vi "Group Terminals.vi"(9 "Terminal Configs":T3[](array[typedef]), 10 "Terminals":refnum<vi>[](array[refnum])) -> (3 "Grouped Terminals":T1)   [LabVIEW 2020, in "FlexBlocks.lvlib"]
uses:
  FlexBlocks.lvlib
  Terminal Config.ctl
  Type Descriptor.ctl
  Terminal Direction.ctl
  Value Mode.ctl
  Special Terminal.ctl
  Terminal Mode.ctl
  Terminal Group.ctl
  Grouped Terminals.ctl
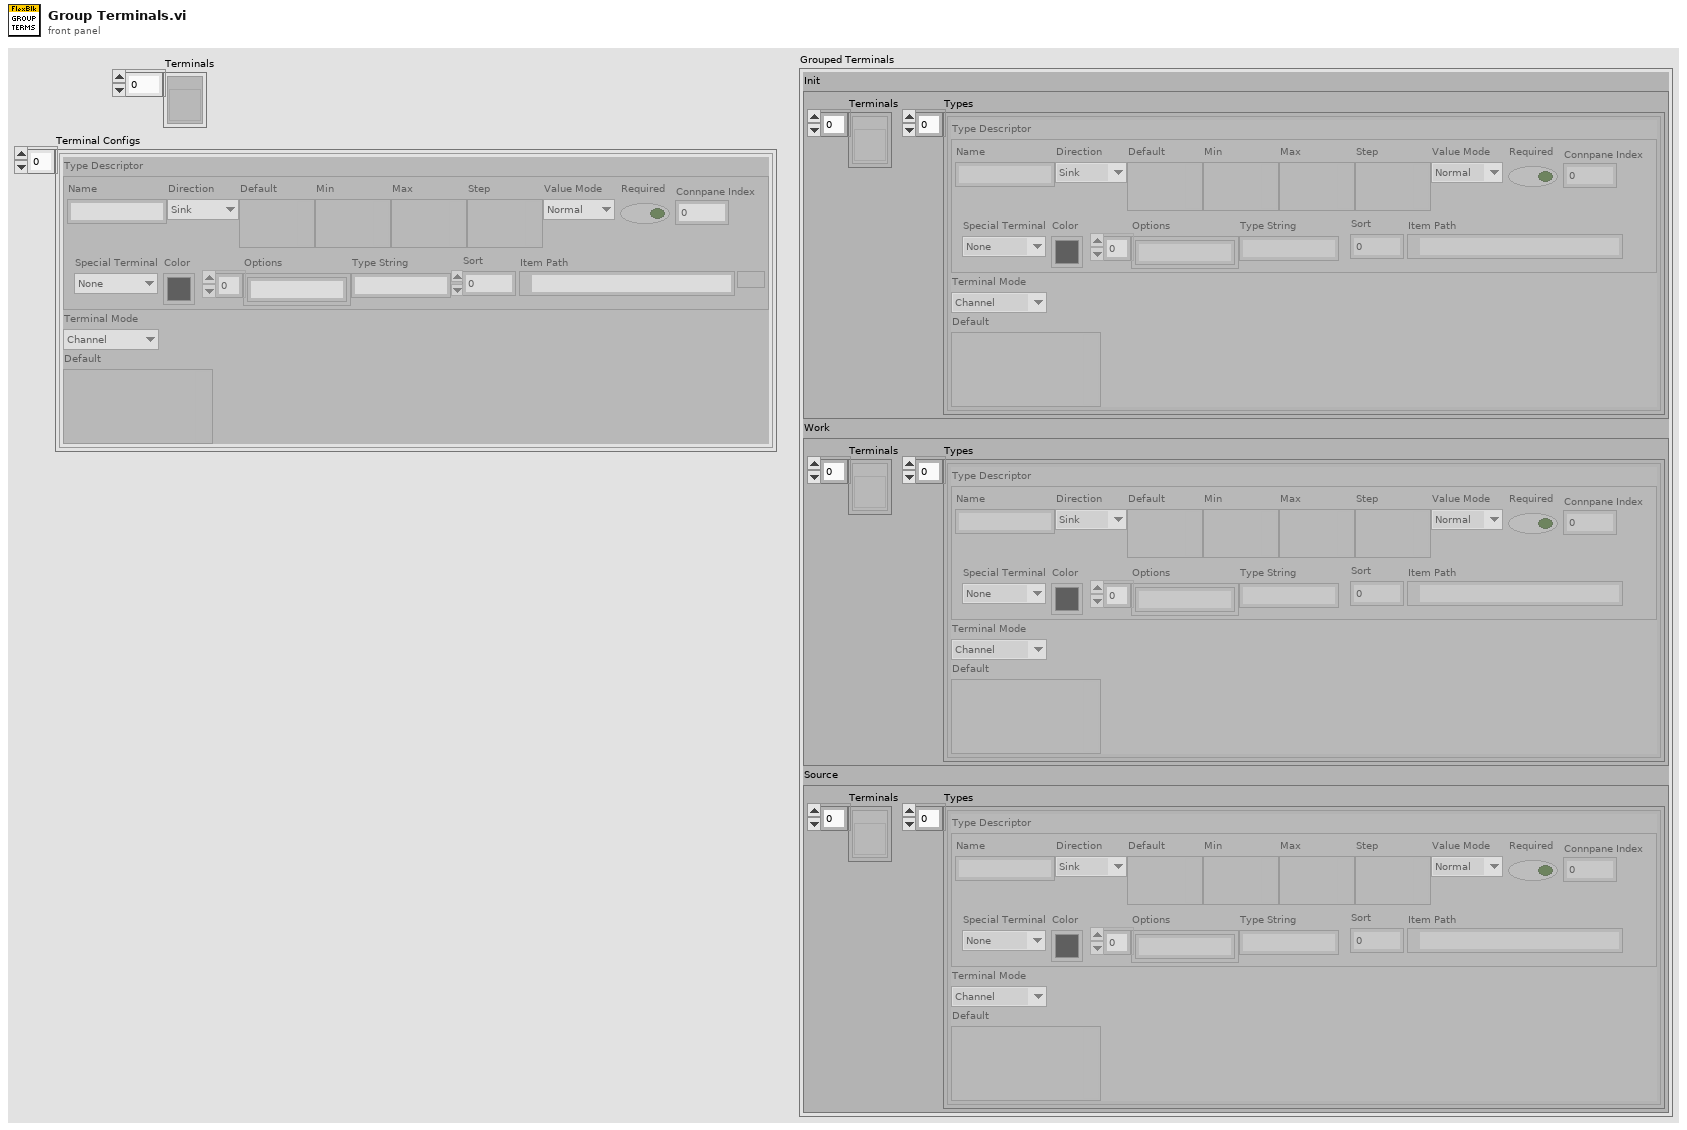
[diagram p1: front panel]
types:
  T1 = typedef "FlexBlocks.lvlib/Grouped Terminals.ctl" = cluster{"Init":T2, "Work":T2, "Source":T2}
  T2 = typedef "FlexBlocks.lvlib/Terminal Group.ctl" = cluster{"Terminals":refnum<vi>[], "Types":T3[]}
  T3 = typedef "FlexBlocks.lvlib/Terminal Config.ctl" = cluster{"Type Descriptor":T4, "Terminal Mode":T8, "Default":variant}
  T4 = typedef "FlexBlocks.lvlib/Type Descriptor.ctl" = cluster{"Name":string, "Direction":T5, "Default":variant, "Min":variant, "Max":variant, "Step":variant, "Value Mode":T6, "Required":bool, "Connpane Index":i32, "Special Terminal":T7, "Color":u32, "Options":string[], "Type String":string, "Sort":i32, "Item Path":path}
  T5 = typedef "FlexBlocks.lvlib/Terminal Direction.ctl" = enum16{"Sink", "Source"}
  T6 = typedef "FlexBlocks.lvlib/Value Mode.ctl" = enum16{"Normal", "Range", "Select"}
  T7 = typedef "FlexBlocks.lvlib/Special Terminal.ctl" = enum16{"None", "Action", "Init", "Tag", "State in", "State out", "Error"}
  T8 = typedef "FlexBlocks.lvlib/Terminal Mode.ctl" = enum16{"Channel", "Config", "Value", "Control Ref"}
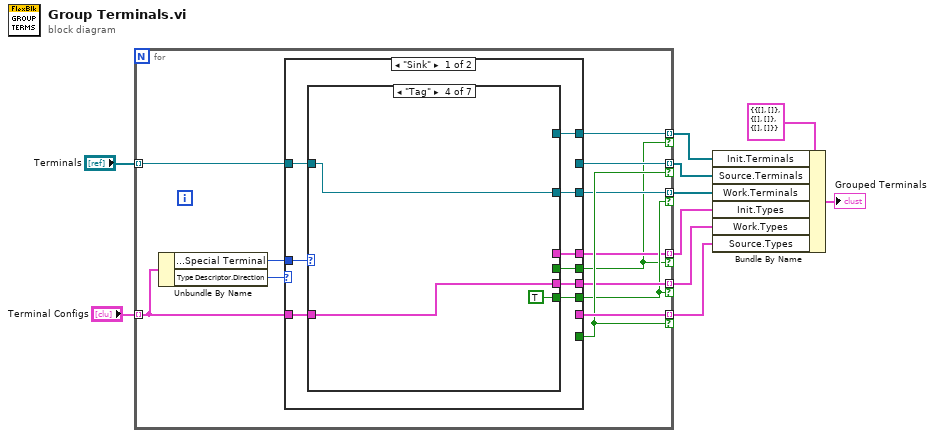
[diagram p0: block diagram]
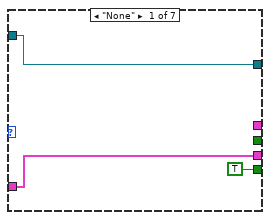
[diagram p2: hidden frame]
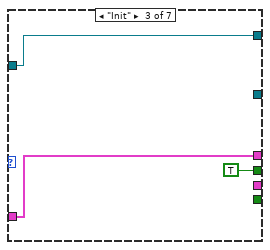
[diagram p4: hidden frame]
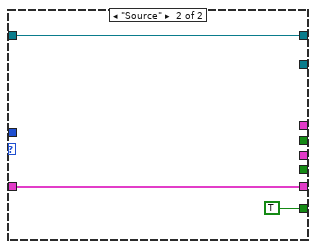
[diagram p8: hidden frame]
diagram:
  n1 = for {
    tunnel: "Terminals" -> [w11] mode=indexing
    tunnel: "Terminal Configs" -> [w21] mode=indexing
    tunnel: [w20] -> w4 mode=indexing if=w18
    tunnel: [w19] -> w3 mode=indexing if=w18
    tunnel: [w17] -> w5 mode=indexing if=w15
    tunnel: [w16] -> w7 mode=indexing if=w15
    tunnel: [w14] -> w2 mode=indexing if=w12
    tunnel: [w13] -> w6 mode=indexing if=w12
    n2 = Unbundle By Name(w21) -> ("Type Descriptor.Special Terminal"=w22:T7, "Type Descriptor.Direction"=w23:T5)
    n3 = case shown="\"Sink\"" w23 {
      tunnel: w22 -> [w32 _]
      tunnel: w11 -> [w31 w42]
      tunnel: w21 -> [w30 w44]
      tunnel: [_ w44] -> w20
      tunnel: [_ TRUE] -> w18
      tunnel: [_ w42] -> w19
      tunnel: [w29 _] -> w17
      tunnel: [w28 _] -> w16
      tunnel: [w27 _] -> w15
      tunnel: [w26 _] -> w14
      tunnel: [w25 _] -> w13
      tunnel: [w24 _] -> w12
      frame "Sink" {
        n4 = case shown="\"Tag\"" w32 {
          tunnel: w31 -> [w34 _ w38 w41 _ _ _]
          tunnel: w30 -> [w35 _ w37 w39 _ _ _]
          tunnel: [w35 _ _ w39 _ _ _] -> w29
          tunnel: [w34 _ _ w41 _ _ _] -> w28
          tunnel: [TRUE _ _ TRUE _ _ _] -> w27
          tunnel: [_ _ w38 _ _ _ _] -> w26
          tunnel: [_ _ w37 _ _ _ _] -> w25
          tunnel: [_ _ TRUE _ _ _ _] -> w24
          frame "None" {
          }
          frame "Action" {
          }
          frame "Init" {
          }
          frame "Tag" {
          }
          frame "State in" {
          }
          frame "State out" {
          }
          frame "Error" {
          }
        }
      }
      frame "Source" {
      }
    }
  }
  n5 = Bundle By Name(cluster=T1 {"Init"={"Terminals"=[], "Types"=[]}, "Work"={"Terminals"=[], "Types"=[]}, "Source"={"Terminals"=[], "Types"=[]}} ("Grouped Terminals"), "Init.Terminals"=w2, "Source.Terminals"=w3, "Work.Terminals"=w7, "Init.Types"=w6, "Work.Types"=w5, "Source.Types"=w4) -> (→"Grouped Terminals":T1)
